vi "GUI_TRA_NEW.vi"() -> ()   [LabVIEW 2013]
uses:
  Device Drivers/TRAServer/StatusTRA_TypDef.ctl
  Shared/GUI_Template/GUI_master/tcp new data cluster.ctl
  General-Controler/firstCall_TypDef.ctl
  Device Drivers/TRAServer/TRAServer.lvclass
panel:
  out "status ref":refnum<vi>[](array[refnum])
  out "pathRef":refnum<vi>[](array[refnum])
  in  "pushSave":bool
  out "Page Label":string="StagingTRA1"
  in  "save::4":bool caption="save"
  in  "save::3":bool caption="save"
  in  "save::2":bool caption="save"
  in  "save::1":bool caption="save"
  in  "LocalSavingPath::4":path=path "Z:/5_resources/StagingResources/TRAposition/testNEW" caption="LocalSavingPath::1"
  in  "LocalSavingPath::3":path=path "Z:/5_resources/StagingResources/TRAposition/testNEW" caption="LocalSavingPath::1"
  in  "LocalSavingPath::2":path=path "Z:/5_resources/StagingResources/TRAposition/testNEW" caption="LocalSavingPath::1"
  in  "LocalSavingPath::1":path=path "Z:/5_resources/StagingResources/TRAposition/testNEW"
  in  "save":bool
  out "GUIdevice 3":string="StagingTRA3"
  out "GUIdevice 4":string="TREX TRA1"
  in  "new":dbl
  out "error out":errorcluster
  out "GUIdevice 2":string="StagingTRA2"
  in  "Tab Control":T1(tab)
  in  "StepSize::1":dbl=0.01 caption="StepSize" min=-1.0 max=1.0 format="%#_2p"
  in  "Cluster 20":T2
  in  "Y":T4={"position::1"=2.74161, "Channel::1"=enum."Axis 2", "Status::1"=enum."DISABLE"} {"position::1" min=0.0 max=6.0 format="%#_8g"}
  in  "X":T5={"position::1"=3.02685, "Channel::1"=enum."Axis 1", "Status::1"=enum."DISABLE"} {"position::1" min=0.0 max=6.0 format="%#_8g"}
  in  "Cluster 40":T6
  in  "Cluster 50":T7
  in  "Cluster 30":T8
  out "device status::1":string="Initialized" caption="Device status"
  in  "<command>::1":bool
  in  "StepSize::2":dbl=0.01 caption="StepSize" min=-1.0 max=1.0 format="%#_2p"
  in  "Cluster 23":T9
  in  "Y":T10={"position::2"=3.24237, "Channel::2"=enum."Axis 2", "Status::2"=enum."DISABLE"} {"position::2" min=0.0 max=0.0 format="%#_8g"}
  in  "X":T11={"position::2"=2.27011, "Channel::2"=enum."Axis 1", "Status::2"=enum."DISABLE"} {"position::2" min=0.0 max=0.0 format="%#_8g"}
  in  "Cluster 43":T12
  in  "Cluster 53":T13
  in  "Cluster 33":T14
  out "device status::2":string="Initialized" caption="Device status"
  in  "<command>::2":bool
  in  "StepSize::3":dbl=0.01 caption="StepSize" min=-1.0 max=1.0 format="%#_2p"
  in  "Cluster 22":T15
  in  "Y":T16={"position::3"=5.00224, "Channel::3"=enum."Axis 2", "Status::3"=enum."DISABLE"} {"position::3" min=0.0 max=0.0 format="%#_8g"}
  in  "X":T17={"position::3"=1.52721, "Channel::3"=enum."Axis 1", "Status::3"=enum."DISABLE"} {"position::3" min=0.0 max=6.0 format="%#_8g"}
  in  "Cluster 42":T18
  in  "Cluster 52":T19
  in  "Cluster 32":T20
  out "device status::3":string="Initialized" caption="Device status"
  in  "<command>::3":bool
  in  "StepSize::4":dbl=0.01 caption="StepSize" min=-1.0 max=1.0 format="%#_2p"
  in  "Cluster 21":T21
  in  "Y":T22={"position::4"=4.68088, "Channel::4"=enum."Axis 2", "Status::4"=enum."DISABLE"} {"position::4" min=0.0 max=0.0 format="%#_8g"}
  in  "X":T23={"position::4"=0.99394, "Channel::4"=enum."Axis 1", "Status::4"=enum."DISABLE"} {"position::4" min=0.0 max=0.0 format="%#_8g"}
  in  "Cluster 41":T24
  in  "Cluster 51":T25
  in  "Cluster 31":T26
  out "device status::4":string="Initialized" caption="Device status"
  in  "<command>::4":bool
  in  "Mirror":T27(ring)
  out "GUIdevice 1":string="StagingTRA1"
  in  "stop":bool=TRUE
  in  "Refresh Button":bool
  out "UDP error message":string
  # "version 1.0.0 (2012/07/27)"
  # "Save All"
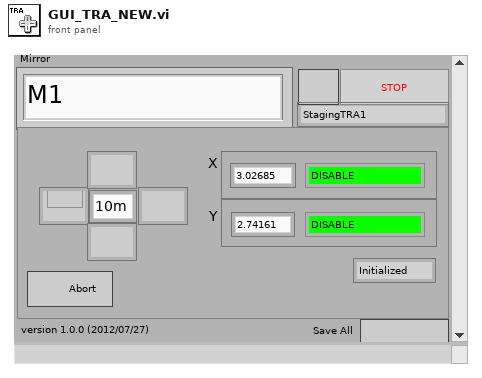
[diagram p1: front panel]
types:
  T1 = enum32{"StagingTRA1", "StagingTRA2", "StagingTRA3", "TREX TRA1"}
  T2 = cluster{"relativeMovePos::1":bool, "Channel::1":enum16{"Axis 1", "Axis 3", "Axis 5"}}
  T3 = typedef "TRAServer.lvclass/StatusTRA_TypDef.ctl" = enum16{"NOT REFERENCED", "CONFIGURATION", "HOMING", "MOVING", "READY", "DISABLE", "JOGGING"}
  T4 = cluster{"position::1":dbl, "Channel::1":enum16{"Axis 2", "Axis 4", "Axis 6"}, "Status::1":T3}
  T5 = cluster{"position::1":dbl, "Channel::1":enum16{"Axis 1", "Axis 3", "Axis 5"}, "Status::1":T3}
  T6 = cluster{"relativeMovePos::1":bool, "Channel::1":enum16{"Axis 2", "Axis 4", "Axis 6"}}
  T7 = cluster{"relativeMoveNeg::1":bool, "Channel::1":enum16{"Axis 2", "Axis 4", "Axis 6"}}
  T8 = cluster{"relativeMoveNeg::1":bool, "Channel::1":enum16{"Axis 1", "Axis 3", "Axis 5"}}
  T9 = cluster{"relativeMovePos::2":bool, "Channel::2":enum16{"Axis 1", "Axis 3", "Axis 5"}}
  T10 = cluster{"position::2":dbl, "Channel::2":enum16{"Axis 2", "Axis 4", "Axis 6"}, "Status::2":T3}
  T11 = cluster{"position::2":dbl, "Channel::2":enum16{"Axis 1", "Axis 3", "Axis 5"}, "Status::2":T3}
  T12 = cluster{"relativeMovePos::2":bool, "Channel::2":enum16{"Axis 2", "Axis 4", "Axis 6"}}
  T13 = cluster{"relativeMoveNeg::2":bool, "Channel::2":enum16{"Axis 2", "Axis 4", "Axis 6"}}
  T14 = cluster{"relativeMoveNeg::2":bool, "Channel::2":enum16{"Axis 1", "Axis 3", "Axis 5"}}
  T15 = cluster{"relativeMovePos::3":bool, "Channel::3":enum16{"Axis 1", "Axis 3", "Axis 5"}}
  T16 = cluster{"position::3":dbl, "Channel::3":enum16{"Axis 2", "Axis 4", "Axis 6"}, "Status::3":T3}
  T17 = cluster{"position::3":dbl, "Channel::3":enum16{"Axis 1", "Axis 3", "Axis 5"}, "Status::3":T3}
  T18 = cluster{"relativeMovePos::3":bool, "Channel::3":enum16{"Axis 2", "Axis 4", "Axis 6"}}
  T19 = cluster{"relativeMoveNeg::3":bool, "Channel::3":enum16{"Axis 2", "Axis 4", "Axis 6"}}
  T20 = cluster{"relativeMoveNeg::3":bool, "Channel::3":enum16{"Axis 1", "Axis 3", "Axis 5"}}
  T21 = cluster{"relativeMovePos::4":bool, "Channel::4":enum16{"Axis 1", "Axis 3", "Axis 5"}}
  T22 = cluster{"position::4":dbl, "Channel::4":enum16{"Axis 2", "Axis 4", "Axis 6"}, "Status::4":T3}
  T23 = cluster{"position::4":dbl, "Channel::4":enum16{"Axis 1", "Axis 3", "Axis 5"}, "Status::4":T3}
  T24 = cluster{"relativeMovePos::4":bool, "Channel::4":enum16{"Axis 2", "Axis 4", "Axis 6"}}
  T25 = cluster{"relativeMoveNeg::4":bool, "Channel::4":enum16{"Axis 2", "Axis 4", "Axis 6"}}
  T26 = cluster{"relativeMoveNeg::4":bool, "Channel::4":enum16{"Axis 1", "Axis 3", "Axis 5"}}
  T27 = enum16{"M1", "BS", "M3", "OAP1", "M4", "OAP2", "M5", "n/a", "n/a ", "M20", "SIM", "M22"}
  T28 = typedef "tcp new data cluster.ctl" = cluster{"EventEnum":enum16{"new data", "connection status update"}, "Device name":string}
  T29 = typedef "firstCall_TypDef.ctl" = enum16{"reset", "read"}
  T30 = typedef "LVFontTypeDef.ctl" = cluster{"Font Name":string, "Size":u16, "Bold":bool, "Italic":bool, "Underline":bool, "Strikeout":bool, "Color":u32}
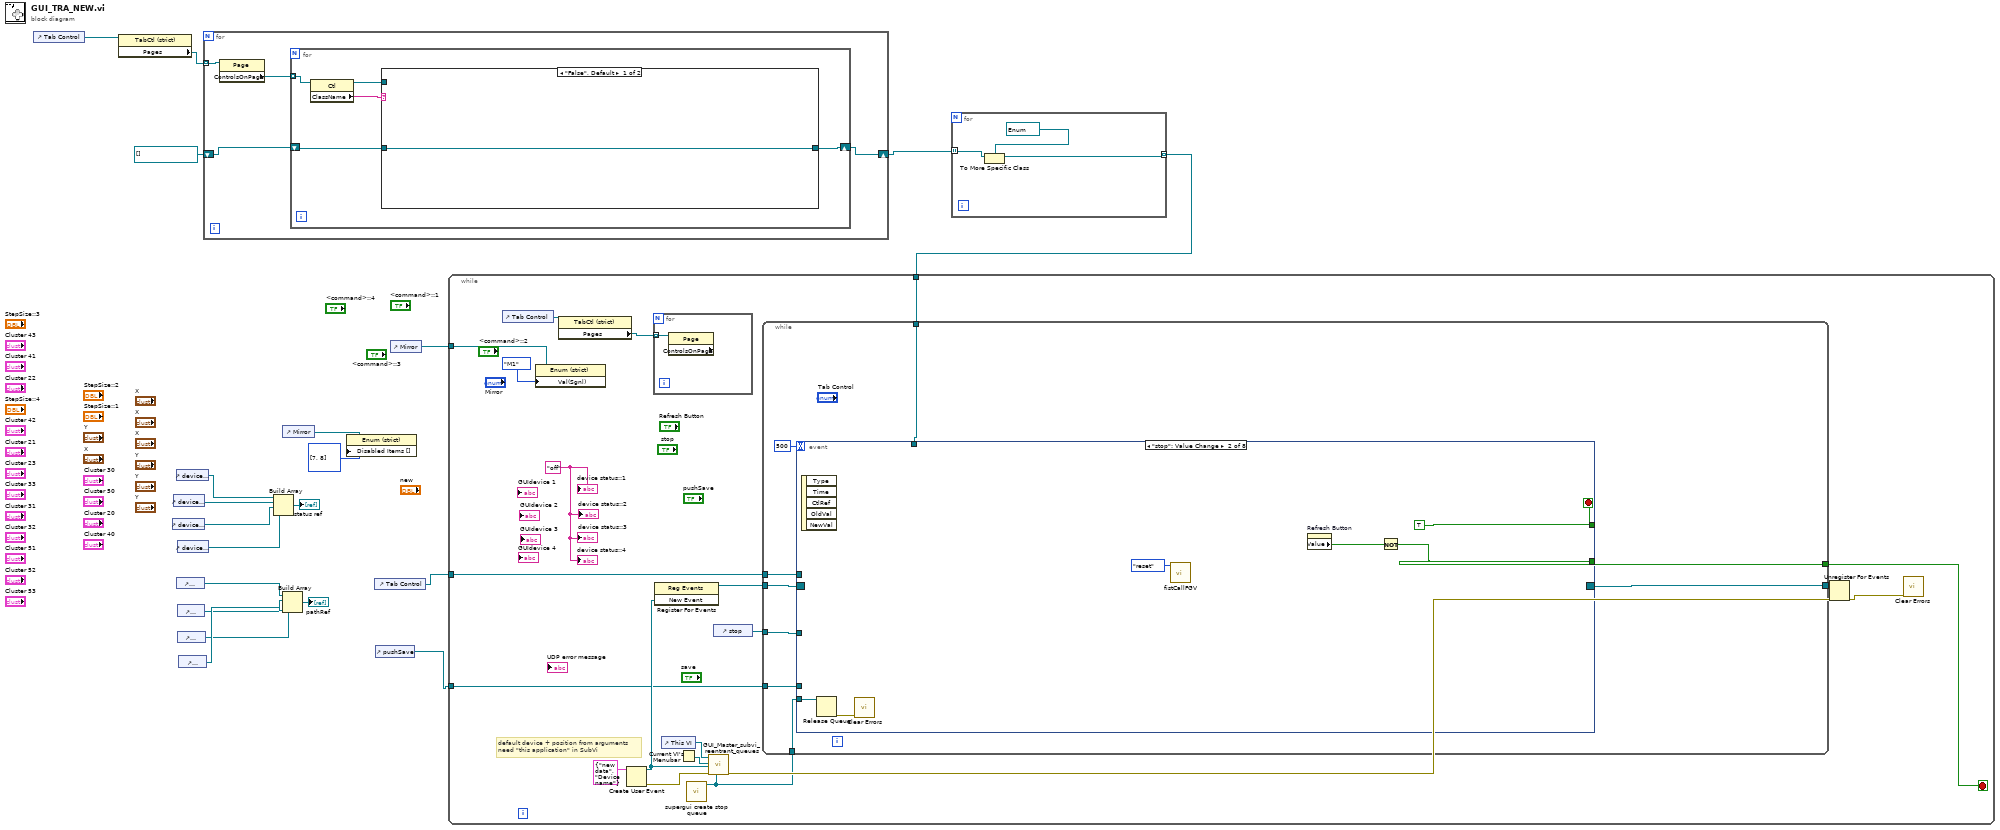
[diagram p0: block diagram]
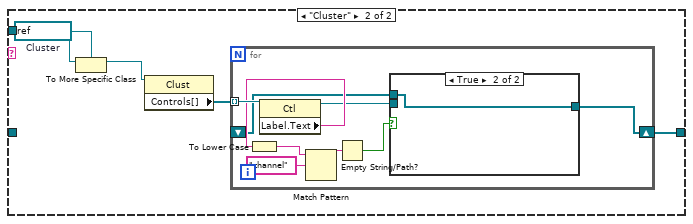
[diagram p2: hidden frame]
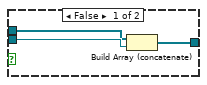
[diagram p3: hidden frame]
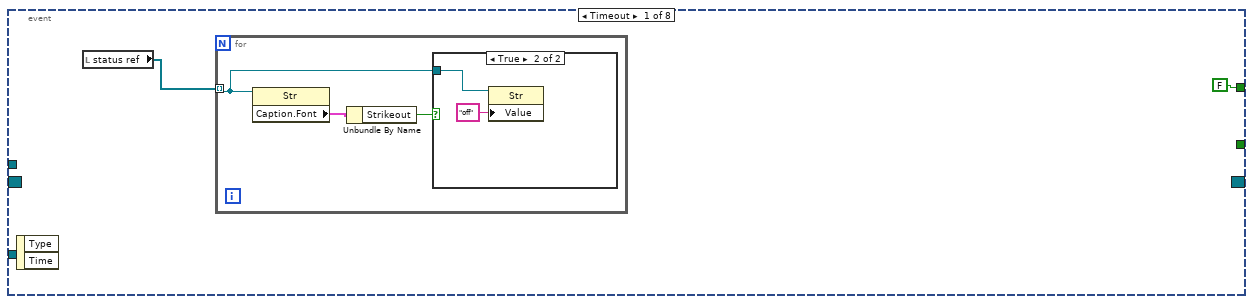
[diagram p4: hidden frame]
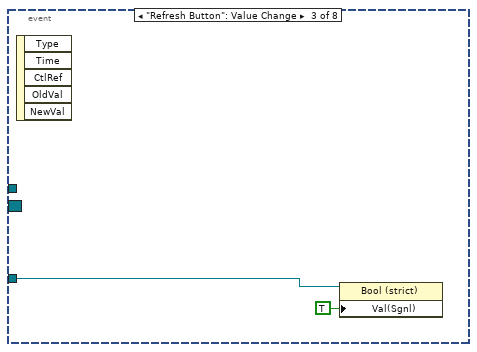
[diagram p6: hidden frame]
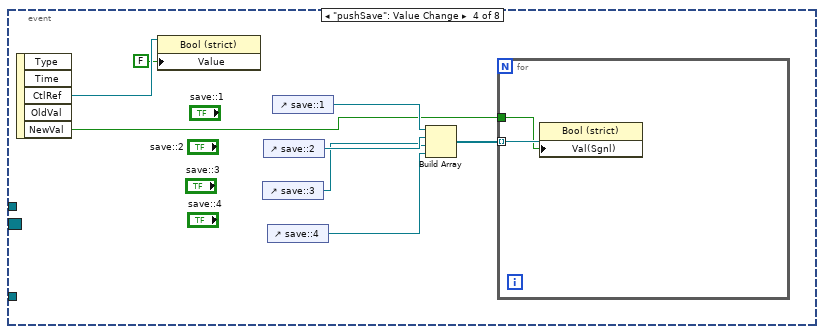
[diagram p7: hidden frame]
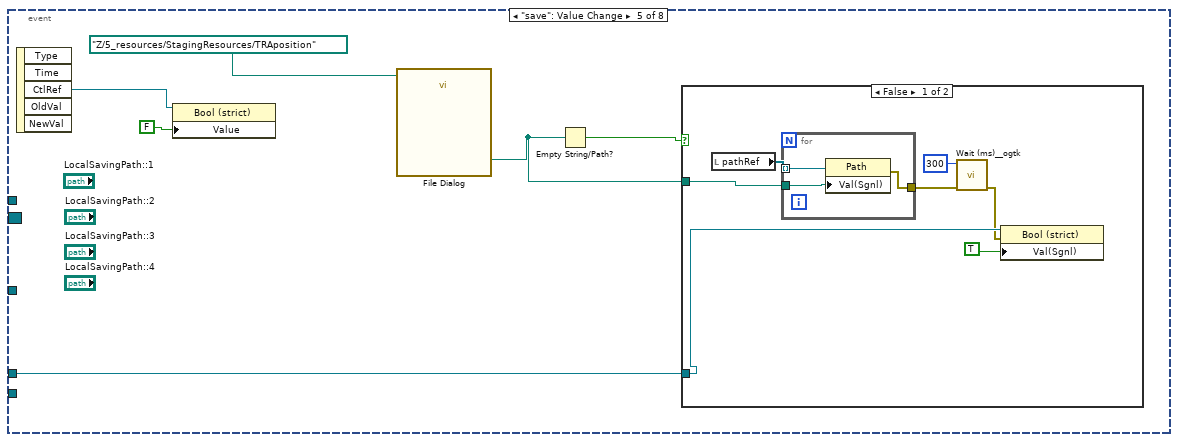
[diagram p8: hidden frame]
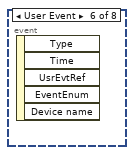
[diagram p10: hidden frame]
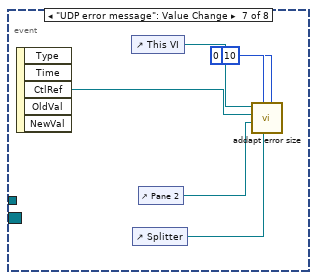
[diagram p11: hidden frame]
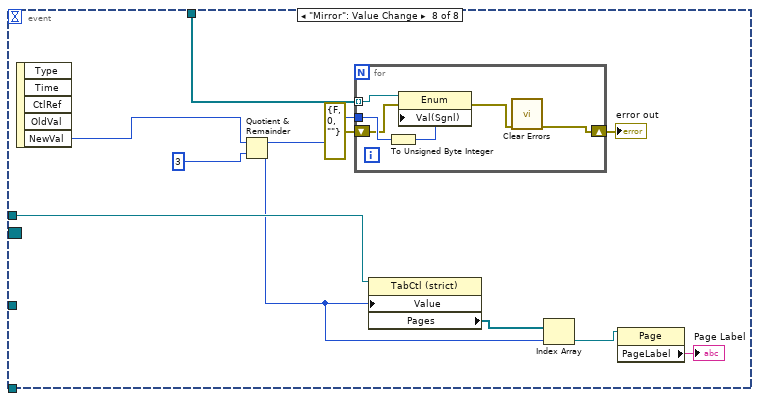
[diagram p12: hidden frame]
diagram:
  n1 = control-ref of="Tab Control"() -> (w20:refnum<vi>)
  n2 = property class="TabCtl (strict)"(reference=w20) -> ("Pages"=w19:refnum<vi>[])  [unwired: 1 in, 2 out]
  n3 = control-ref of="device status::3"() -> (w3:refnum<vi>)
  n4 = control-ref of="device status::2"() -> (w4:refnum<vi>)
  n5 = control-ref of="device status::1"() -> (w5:refnum<vi>)
  n6 = control-ref of="LocalSavingPath::1"() -> (w8:refnum<vi>)
  n7 = control-ref of="device status::4"() -> (w2:refnum<vi>)
  n8 = control-ref of="LocalSavingPath::2"() -> (w9:refnum<vi>)
  n9 = control-ref of="LocalSavingPath::3"() -> (w10:refnum<vi>)
  n10 = control-ref of="LocalSavingPath::4"() -> (w11:refnum<vi>)
  n11 = for {
    tunnel: w19 -> [w24] mode=indexing
    shift-right: [w22] -> w17
    shift-left: refnum<vi>[] [] -> [w21]
    n12 = property class="Page"(reference=w24) -> ("ControlsOnPage"=w23:refnum<vi>[])  [unwired: 1 in, 2 out]
    n13 = for {
      tunnel: w23 -> [w29] mode=indexing
      shift-right: [w26] -> w22
      shift-left: w21 -> [w25]
      n14 = property class="Ctl"(reference=w29) -> (reference out=w27:refnum<vi>, "ClassName"=w28:string)  [unwired: 1 in, 1 out]
      n15 = case shown="\"False\", Default" w28 {
        tunnel: w27 -> [_ w35]
        tunnel: [w30 w31] -> w26
        tunnel: w25 -> [w30 _]
        frame "False", Default {
        }
        frame "Cluster" {
          w34 = refnum<vi> refnum  # Cluster
          n16 = To More Specific Class(target class=w34, reference=w35) -> (specific class reference=w33:refnum<vi>)  [unwired: 1 in, 1 out]
          n17 = property class="Clust"(reference=w33) -> ("Controls[]"=w32:refnum<vi>[])  [unwired: 1 in, 2 out]
          n18 = for {
            tunnel: w32 -> [w44] mode=indexing
            shift-right: [w37] -> w31
            shift-left: _ -> [w36]
            n19 = property class="Ctl"(reference=w44) -> (reference out=w38:refnum<vi>, "Label.Text"=w42:string)  [unwired: 1 in, 1 out]
            n20 = To Lower Case(string=w42) -> (all lower case string=w41:string)
            n21 = Match Pattern(string=w41, regular expression="channel") -> (match substring=w40:string)  [unwired: 1 in, 3 out]
            n22 = Empty String/Path?(string/path=w40) -> (empty?=w39:bool)
            n23 = case shown="True" w39 {
              tunnel: w38 -> [w47 _]
              tunnel: [w46 w48] -> w37
              tunnel: w36 -> [w45 w48]
              frame False {
                n24 = Build Array (concatenate)(w45, w47) -> (w46:refnum<vi>[])
              }
              frame True {
              }
            }
          }
        }
      }
    }
  }
  n25 = Build Array(w5, w4, w3, w2) -> (→"status ref":refnum<vi>[])
  n26 = control-ref of="Mirror"() -> (w13:refnum<vi>)
  n27 = Build Array(w8, w9, w10, w11) -> (→"pathRef":refnum<vi>[])
  n28 = property class="Enum (strict)"(reference=w13, "Disabled Items []"=i32[] [7, 8]) -> ()  [unwired: 1 in, 2 out]
  n29 = control-ref of="Tab Control"() -> (w15:refnum<vi>)
  n30 = control-ref of="pushSave"() -> (w6:refnum<vi>)
  n31 = control-ref of="Mirror"() -> (w12:refnum<vi>)
  n32 = for {
    tunnel: w17 -> [w51] mode=indexing
    tunnel: [w50] -> w16 mode=indexing
    n33 = To More Specific Class(target class=refnum<vi> refnum ("Channel::2"), reference=w51) -> (specific class reference=w50:refnum<vi>)  [unwired: 1 in, 1 out]
  }
  n34 = while {
    tunnel: w16 -> [w58]
    tunnel: w15 -> [w57]
    tunnel: w12 -> [w56]
    tunnel: w6 -> [w54]
    stop <- w69 stop-if-true
    w53 = "off" ("device status::1")
    # "default device + position from arguments\nneed \"this application\" in SubVi"
    n35 = control-ref of="Tab Control"() -> (w60:refnum<vi>)
    n36 = property class="Enum (strict)"(reference=w56, "Val(Sgnl)"=T27."M1" ("Value (Signaling)")) -> ()  [unwired: 1 in, 2 out]
    n37 = property class="TabCtl (strict)"(reference=w60) -> ("Pages"=w59:refnum<vi>[])  [unwired: 1 in, 2 out]
    n38 = Create User Event(user event datatype=T28 {"EventEnum"=enum."new data", "Device name"="Device name"} ("New Event")) -> (user event=w63:refnum<user-event>, error out=w64:errorcluster)  [unwired: 1 in]
    n39 = for {
      tunnel: w59 -> [w72] mode=indexing
      n40 = property class="Page" props=["ControlsOnPage"](reference=w72) -> ()  [unwired: 1 in, 3 out]
    }
    n41 = register-events(w63) -> (reference out=w71:refnum<event-registration>)  [unwired: 2 in, 1 out]
    n42 = control-ref of="This VI"() -> (w67:refnum<vi>)
    n43 = Current VI's Menubar() -> (w66:refnum<k9>)
    n44 = call "supergui create stop queue.vi"() -> ("STOP Queue out"=w52:refnum<queue>)  [unwired: 11 in]
    n45 = call "GUI_Master_subvi_reentrant_queues.vi"("STOP Queue in"=w52, "error in (no error)"=w64, "tcp data event"=w63, "Caller menu reference"=w66, "Caller VI ref"=w67) -> ("error out"=w62:errorcluster)  [unwired: 6 in]
    n46 = control-ref of="stop"() -> (w68:refnum<vi>)
    n47 = while {
      tunnel: w71 -> [w82]
      tunnel: [w81] -> w70
      tunnel: [w79] -> w69
      tunnel: w68 -> [w78]
      tunnel: w58 -> [w77]
      tunnel: w57 -> [w76]
      tunnel: w54 -> [w75]
      tunnel: w52 -> [w73]
      stop <- w80 stop-if-true
      n48 = event shown="[1] \"stop\": Value Change" {
        selector: w82 -> [_ _ _ _ _ _ _ _]
        dyn-events: [_ _ _ _ _ _ _ _] -> w81
        timeout: 500 -> [_ _ _ _ _ _ _ _]
        tunnel: [FALSE TRUE _ _ _ _ _ _] -> w80
        tunnel: [_ w93 _ _ _ _ _ _] -> w79
        tunnel: w78 -> [_ _ w97 _ _ _ _ _]
        tunnel: w77 -> [_ _ _ _ _ _ _ w140]
        tunnel: w76 -> [_ _ _ _ _ _ _ w134]
        tunnel: w75 -> [_ _ _ _ w110 _ _ _]
        tunnel: w73 -> [_ w90 _ _ _ _ _ _]
        event Timeout {
          n49 = event-data() -> ()  [unwired: 1 in, 2 out]
          n50 = local read "status ref"() -> (w83:refnum<vi>[])
          n51 = for {
            tunnel: w83 -> [w85] mode=indexing
            n52 = property class="Str"(reference=w85) -> ("Caption.Font"=w87:T30)  [unwired: 1 in, 2 out]
            n53 = Unbundle By Name(w87) -> ("Strikeout"=w86:bool)
            n54 = case shown="True" w86 {
              tunnel: w85 -> [_ w89]
              frame False {
              }
              frame True {
                n55 = property class="Str"(reference=w89, "Value"="off") -> ()  [unwired: 1 in, 2 out]
              }
            }
          }
        }
        event "stop": Value Change {
          n56 = event-data() -> ()  [unwired: 1 in, 5 out]
          n57 = Release Queue(queue=w90) -> (error out=w91:errorcluster)  [unwired: 2 in, 2 out]
          n58 = call <vilib>:"Clear Errors.vi"("error in (no error)"=w91) -> ()  [unwired: 6 in, 1 out]
          n59 = call "fistCallFGV.vi"("Function"=firstCall_TypDef."reset") -> ()  [unwired: 9 in, 2 out]
          n60 = property on="Refresh Button" class="Bool (strict)"() -> ("Value"=w94:bool)  [unwired: 2 in, 2 out]
          n61 = Not(x=w94) -> (.not. x?=w93:bool)
        }
        event "Refresh Button": Value Change {
          n62 = event-data() -> ()  [unwired: 1 in, 5 out]
          n63 = property class="Bool (strict)"(reference=w97, "Val(Sgnl)"=TRUE ("Value (Signaling)")) -> ()  [unwired: 1 in, 2 out]
        }
        event "pushSave": Value Change {
          n64 = event-data() -> ("CtlRef"=w99:refnum<vi>, "NewVal"=w100:bool)  [unwired: 1 in, 3 out]
          n65 = property class="Bool (strict)"(reference=w99, "Value"=FALSE) -> ()  [unwired: 1 in, 2 out]
          n66 = control-ref of="save::3"() -> (w103:refnum<vi>)
          n67 = control-ref of="save::2"() -> (w104:refnum<vi>)
          n68 = control-ref of="save::4"() -> (w102:refnum<vi>)
          n69 = control-ref of="save::1"() -> (w105:refnum<vi>)
          n70 = Build Array(w105, w104, w103, w102) -> (w101:refnum<vi>[])
          n71 = for {
            tunnel: w101 -> [w107] mode=indexing
            tunnel: w100 -> [w106]
            n72 = property class="Bool (strict)"(reference=w107, "Val(Sgnl)"=w106) -> ()  [unwired: 1 in, 2 out]
          }
        }
        event "save": Value Change {
          n73 = event-data() -> ("CtlRef"=w109:refnum<vi>)  [unwired: 1 in, 4 out]
          n74 = property class="Bool (strict)"(reference=w109, "Value"=FALSE) -> ()  [unwired: 1 in, 2 out]
          n75 = call "File Dialog"("start path"=path "Z:/5_resources/StagingResources/TRAposition") -> ("selected path"=w112:path)  [unwired: 11 in, 3 out]
          n76 = Empty String/Path?(string/path=w112) -> (empty?=w111:bool)
          n77 = case shown="False" w111 {
            tunnel: w112 -> [w120 _]
            tunnel: w110 -> [w116 _]
            frame False {
              n78 = local read "pathRef"() -> (w119:refnum<vi>[])
              n79 = for {
                tunnel: w119 -> [w123] mode=indexing
                tunnel: w120 -> [w122]
                tunnel: [w121] -> w118
                n80 = property class="Path"(reference=w123, "Val(Sgnl)"=w122) -> (error out=w121:errorcluster)  [unwired: 1 in, 1 out]
              }
              n81 = call <userlib>:"Wait (ms)__ogtk.vi"("error in (no error)"=w118, "milliseconds to wait"=u32 300) -> ("error out"=w115:errorcluster)  [unwired: 8 in, 1 out]
              n82 = property class="Bool (strict)"(reference=w116, error in=w115, "Val(Sgnl)"=TRUE) -> ()  [unwired: 2 out]
            }
            frame True {
            }
          }
        }
        event User Event {
          n83 = event-data() -> ()  [unwired: 1 in, 5 out]
        }
        event "UDP error message": Value Change {
          n84 = event-data() -> ("CtlRef"=w129:refnum<vi>)  [unwired: 1 in, 4 out]
          n85 = control-ref of="This VI"() -> (w128:refnum<vi>)
          n86 = control-ref of="Splitter"() -> (w125:refnum<vi>)
          n87 = control-ref of="Pane 2"() -> (w124:refnum<vi>)
          n88 = call "addapt error size.vi"("stepsize"=10, "Splitter"=w125, "milliseconds to wait"=u32 0, "Pane in"=w124, "String"=w129, "VI in"=w128) -> ()  [unwired: 6 in]
        }
        event "Mirror": Value Change {
          n89 = event-data() -> ("NewVal"=w139:T27)  [unwired: 1 in, 4 out]
          n90 = Quotient & Remainder(x=w139, y=3) -> (x-y*floor(x/y)=w137:i32, floor(x/y)=w132:i32)
          n91 = for {
            tunnel: w140 -> [w146] mode=indexing
            tunnel: w137 -> [w144]
            shift-right: [w142] -> w135
            shift-left: errorcluster {"status"=FALSE, "code"=0, "source"=""} ("error out") -> [w141]
            n92 = To Unsigned Byte Integer(number=w144) -> (unsigned 8bit integer=w143:u8)
            n93 = property class="Enum"(reference=w146, error in=w141, "Val(Sgnl)"=w143) -> (error out=w145:errorcluster)  [unwired: 1 out]
            n94 = call <vilib>:"Clear Errors.vi"("error in (no error)"=w145) -> ("error out"=w142:errorcluster)  [unwired: 6 in]
          }
          "error out" <- w135
          n95 = property class="TabCtl (strict)"(reference=w134, "Value"=w132) -> ("Pages"=w133:refnum<vi>[])  [unwired: 1 in, 2 out]
          n96 = Index Array(array=w133, index=w132) -> (element=w131:refnum<vi>)
          n97 = property class="Page"(reference=w131) -> ("PageLabel"=→"Page Label":string)  [unwired: 1 in, 2 out]
        }
      }
    }
    n98 = Unregister For Events(event registration refnum=w70, error in=w62) -> (error out=w61:errorcluster)
    n99 = call <vilib>:"Clear Errors.vi"("error in (no error)"=w61) -> ()  [unwired: 6 in, 1 out]
    "device status::1" <- w53
    "device status::2" <- w53
    "device status::3" <- w53
    "device status::4" <- w53
  }
